vi "Get LakeShore 370 Resistance_VISA.vi"(6 "Read temperature":bool, 7 "Read heater":bool, 8 "error in (no error)":errorcluster, 9 "Seconds between samples":dbl=1.0 format="%_4f", 10 "Channels to scan (empty = don't use scanner option)":i32[](array[numeric]), 11 "VISA resource name":refnum<visa-resource-name>) -> (0 "error out":errorcluster, 2 "Resistance":dbl[](array[numeric]) format="%#_6p", 3 "VISA resource name out":refnum<visa-resource-name>)   [LabVIEW 2015]
uses:
  GPIB/VISA  Send Receive.vi
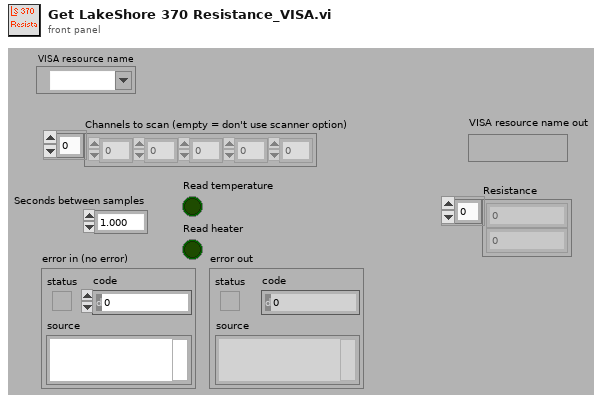
[diagram p1: front panel]
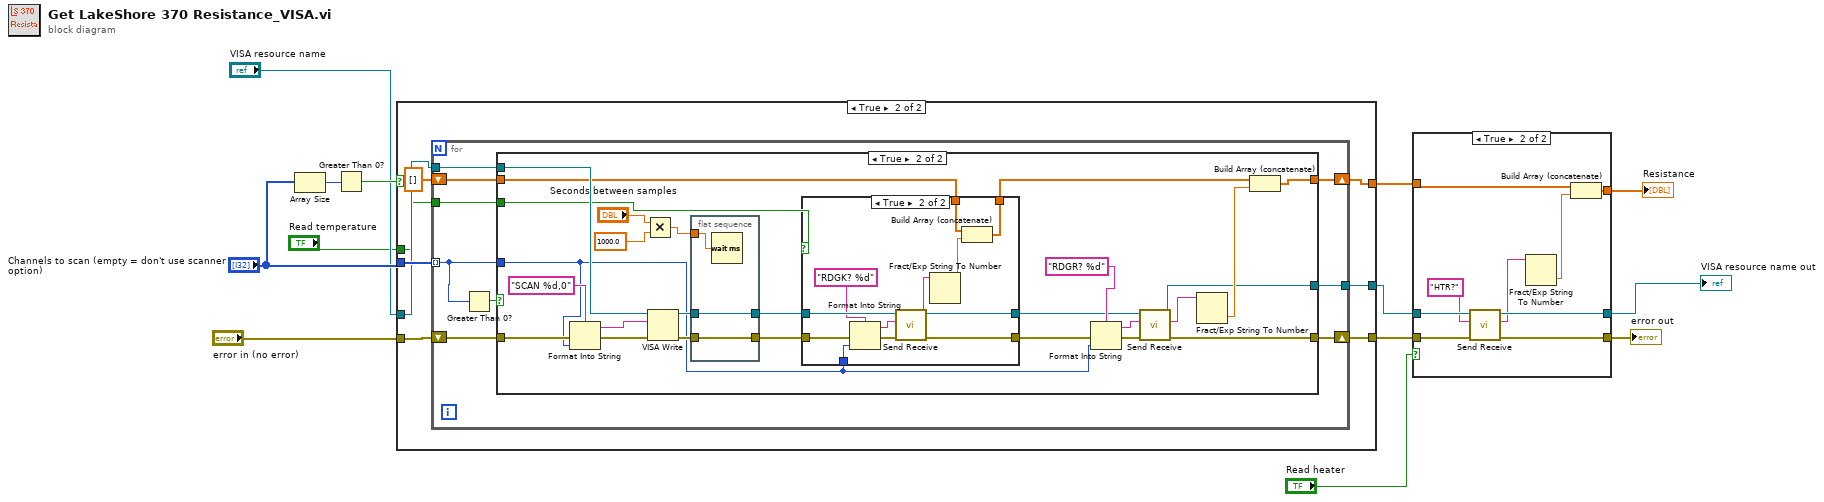
[diagram p0: block diagram]
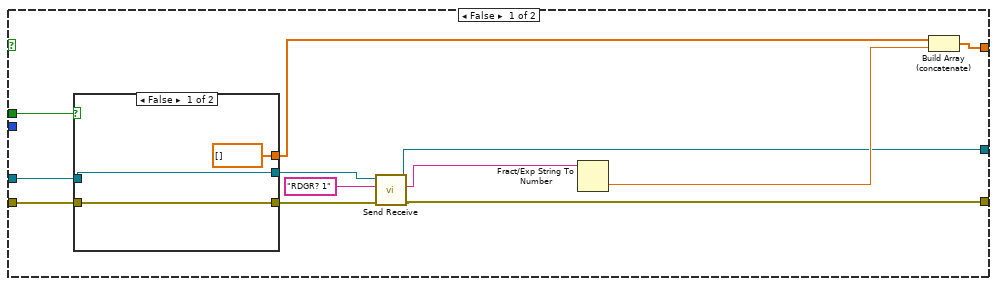
[diagram p3: hidden frame]
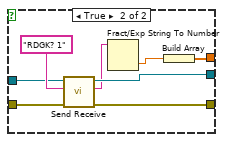
[diagram p4: hidden frame]
diagram:
  n1 = Array Size(array="Channels to scan (empty = don't use scanner option)") -> (size(s)=w13:i32)
  n2 = Greater Than 0?(x=w13) -> (x > 0?=w12:bool)
  n3 = case shown="True" w12 {
    tunnel: "Channels to scan (empty = don't use scanner option)" -> [_ w44]
    tunnel: [w25 w43] -> w3
    tunnel: "error in (no error)" -> [w19 w42]
    tunnel: [w22 w41] -> w7
    tunnel: "VISA resource name" -> [w16 w39]
    tunnel: [w20 w38] -> w5
    tunnel: "Read temperature" -> [w17 w37]
    frame False {
      n4 = case shown="False" w17 {
        tunnel: w19 -> [w28 w36]
        tunnel: [w28 w35] -> w18
        tunnel: w16 -> [w27 w33]
        tunnel: [w27 w32] -> w15
        tunnel: [dbl[] [] w29] -> w14
        frame False {
        }
        frame True {
          n5 = call-poly "Send Receive.vi"("error in (no error)"=w36, "data string in"="RDGK? 1", "VISA Resource Name"=w33) -> ("error out"=w35:errorcluster, "data string out"=w31:string, "VISA Resource Name Out"=w32:refnum<visa-resource-name>)  [unwired: 6 in]
          n6 = Fract/Exp String To Number(string=w31) -> (number=w30:dbl)  [unwired: 4 out]
          n7 = Build Array(w30) -> (w29:dbl[])
        }
      }
      n8 = call-poly "Send Receive.vi"("error in (no error)"=w18, "data string in"="RDGR? 1", "VISA Resource Name"=w15) -> ("error out"=w22:errorcluster, "data string out"=w24:string, "VISA Resource Name Out"=w20:refnum<visa-resource-name>)  [unwired: 6 in]
      n9 = Fract/Exp String To Number(string=w24) -> (number=w21:dbl)  [unwired: 4 out]
      n10 = Build Array (concatenate)(w14, w21) -> (w25:dbl[])
    }
    frame True {
      n11 = for {
        tunnel: w44 -> [w47] mode=indexing
        shift-right: [w50] -> w43
        shift-left: dbl[] [] -> [w49]
        shift-right: [w51] -> w41
        shift-left: w42 -> [w53]
        tunnel: w39 -> [w48]
        tunnel: [w46] -> w38
        tunnel: w37 -> [w45]
        n12 = Greater Than 0?(x=w47) -> (x > 0?=w52:bool)
        n13 = case shown="True" w52 {
          tunnel: w47 -> [_ w57]
          tunnel: w53 -> [w55 w69]
          tunnel: [w55 w75] -> w51
          tunnel: [w56 w79] -> w50
          tunnel: w49 -> [w56 w59]
          tunnel: w48 -> [w54 w71]
          tunnel: [w54 w65] -> w46
          tunnel: w45 -> [_ w60]
          frame False {
          }
          frame True {
            n14 = Format Into String(format string="SCAN %d,0", error in=w69, w57) -> (resulting string=w70:string, error out=w68:errorcluster)  [unwired: 1 in]
            n15 = Multiply(x="Seconds between samples", y=1000.0) -> (x*y=w80:dbl)
            n16 = VISA Write(VISA resource name=w71, write buffer=w70, error in (no error)=w68) -> (VISA resource name out=w67:refnum<visa-resource-name>, error out=w77:errorcluster)  [unwired: 1 out]
            n17 = flat-sequence {
              tunnel: [w99] -> w64
              tunnel: w80 -> [w100]
              tunnel: w77 -> [w99]
              tunnel: w67 -> [w98]
              tunnel: [w98] -> w62
              frame #0 {
                n18 = Wait (ms)(milliseconds to wait=w100) -> ()  [unwired: 1 out]
              }
            }
            n19 = case shown="True" w60 {
              tunnel: w64 -> [w85 w90]
              tunnel: [w85 w97] -> w63
              tunnel: w62 -> [w84 w96]
              tunnel: [w84 w95] -> w61
              tunnel: w59 -> [w83 w93]
              tunnel: [w83 w91] -> w58
              tunnel: w57 -> [_ w87]
              frame False {
              }
              frame True {
                n20 = Format Into String(format string="RDGK? %d" ("data string in"), error in=w90, w87) -> (resulting string=w86:string, error out=w89:errorcluster)  [unwired: 1 in]
                n21 = call-poly "Send Receive.vi"("error in (no error)"=w89, "data string in"=w86, "VISA Resource Name"=w96) -> ("error out"=w97:errorcluster, "data string out"=w94:string, "VISA Resource Name Out"=w95:refnum<visa-resource-name>)  [unwired: 6 in]
                n22 = Fract/Exp String To Number(string=w94) -> (number=w92:dbl)  [unwired: 4 out]
                n23 = Build Array (concatenate)(w93, w92) -> (w91:dbl[])
              }
            }
            n24 = Format Into String(format string="RDGR? %d" ("data string in"), error in=w63, w57) -> (resulting string=w74:string, error out=w66:errorcluster)  [unwired: 1 in]
            n25 = call-poly "Send Receive.vi"("error in (no error)"=w66, "data string in"=w74, "VISA Resource Name"=w61) -> ("error out"=w75:errorcluster, "data string out"=w76:string, "VISA Resource Name Out"=w65:refnum<visa-resource-name>)  [unwired: 6 in]
            n26 = Fract/Exp String To Number(string=w76) -> (number=w72:dbl)  [unwired: 4 out]
            n27 = Build Array (concatenate)(w58, w72) -> (w79:dbl[])
          }
        }
      }
    }
  }
  n28 = case shown="True" "Read heater" {
    tunnel: w7 -> [w102 w112]
    tunnel: [w102 w111] -> w6
    tunnel: w5 -> [w101 w110]
    tunnel: [w101 w109] -> w4
    tunnel: w3 -> [w103 w107]
    tunnel: [w103 w105] -> w2
    frame False {
    }
    frame True {
      n29 = call-poly "Send Receive.vi"("error in (no error)"=w112, "data string in"="HTR?", "VISA Resource Name"=w110) -> ("error out"=w111:errorcluster, "data string out"=w108:string, "VISA Resource Name Out"=w109:refnum<visa-resource-name>)  [unwired: 6 in]
      n30 = Fract/Exp String To Number(string=w108) -> (number=w106:dbl)  [unwired: 4 out]
      n31 = Build Array (concatenate)(w107, w106) -> (w105:dbl[])
    }
  }
  "error out" <- w6
  "Resistance" <- w2
  "VISA resource name out" <- w4
